vi "Iterate On DB Channels.vi"(8 "error out":errorcluster, 11 "board config handle":u32) -> (0 "error IO":errorcluster, 2 "channels":T1 {"speed" items=["OWL429_HIGH_SPEED_CHANNEL", "OWL429_LOW_SPEED_CHANNEL"]; "Labels"."scheduleBuildUnit" items=["Millisecond", "Microsecond"]}, 3 "board config handle":u32)   [LabVIEW 2016]
uses:
  Controls/AIT_Channel Array.ctl
  Controls/Ballard_Channel.ctl
  Controls/AIT_Label.ctl
  Controls/AIT_Word.ctl
  Controls/ARINCParam.ctl
  Shared/Controls and Global/TransferType.ctl
  Controls/Channel_direction.ctl
  Controls/Channel Speed.ctl
  <userlib>/ARINC-429/Owl429.lvlib
  Ballard Arinc-429 System Explorer.lvlib
  Shared/Ballard Arinc-429 Shared.lvlib
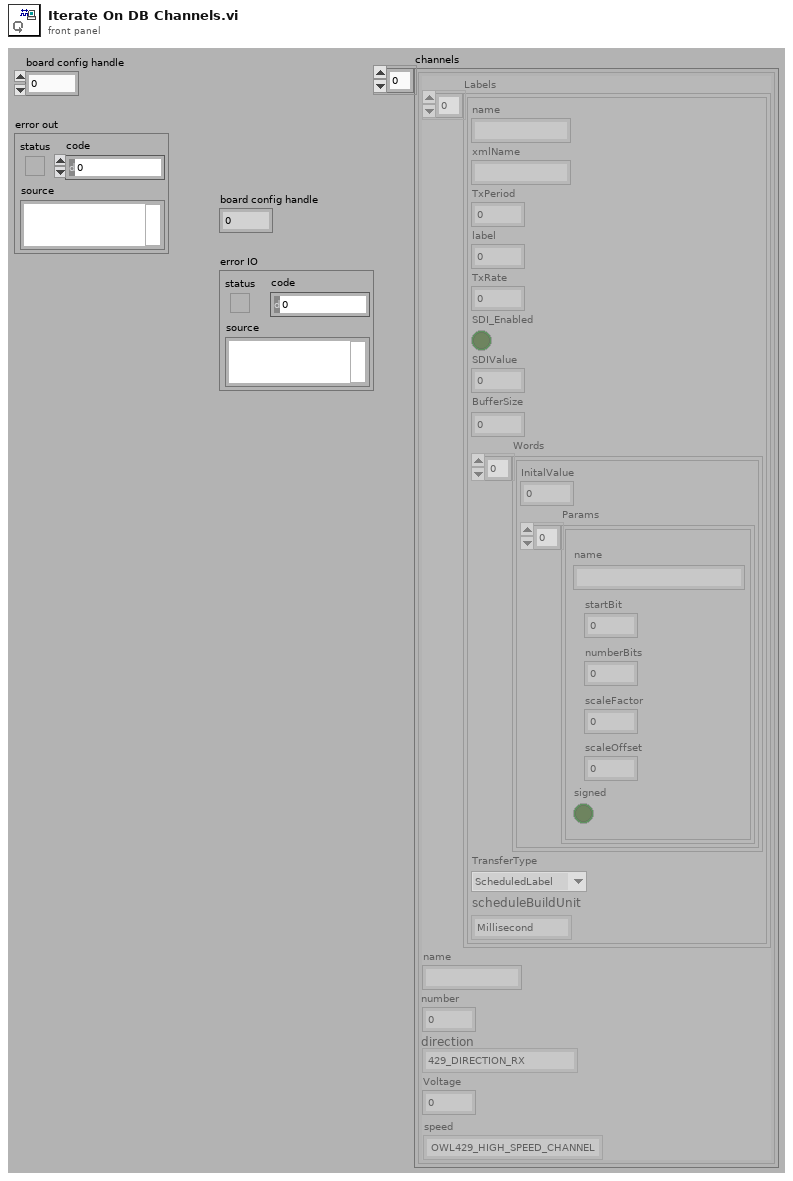
[diagram p1: front panel]
types:
  T1 = typedef "Ballard Arinc-429 System Explorer.lvlib/AIT_Channel Array.ctl" = T2[]
  T2 = typedef "Ballard Arinc-429 System Explorer.lvlib/Ballard_Channel.ctl" = cluster{"Labels":T3[], "name":string, "number":u8, "direction":T7, "Voltage":dbl, "speed":T8}
  T3 = typedef "Ballard Arinc-429 System Explorer.lvlib/AIT_Label.ctl" = cluster{"name":string, "xmlName":string, "TxPeriod":u32, "label":u32, "TxRate":dbl, "SDI_Enabled":bool, "SDIValue":u8, "BufferSize":u32, "Words":T4[], "TransferType":T6, "scheduleBuildUnit":i32}
  T4 = typedef "Ballard Arinc-429 System Explorer.lvlib/AIT_Word.ctl" = cluster{"InitalValue":u32, "Params":T5[]}
  T5 = typedef "Ballard Arinc-429 System Explorer.lvlib/ARINCParam.ctl" = cluster{"name":string, "startBit":i32, "numberBits":i32, "scaleFactor":dbl, "scaleOffset":dbl, "signed":bool}
  T6 = typedef "Ballard Arinc-429 Shared.lvlib/TransferType.ctl" = enum16{"ScheduledLabel", "Acyclic", "Block", "Strobe"}
  T7 = typedef "Channel_direction.ctl" = enum16{"429_DIRECTION_RX", "429_DIRECTION_TX"}
  T8 = typedef "Channel Speed.ctl" = i32
  T9 = enum32{"OWL429_DIRECTION_RX", "OWL429_DIRECTION_TX"}
  T10 = typedef "AIT 429 System Explorer.lvlib/AIT_Channel Array.ctl" = T11[]
  T11 = typedef "AIT 429 System Explorer.lvlib/AIT_Channel.ctl" = cluster{"Labels":T12[], "name":string, "number":u8, "direction":enum16{"OWL429_DIRECTION_RX", "OWL429_DIRECTION_TX"}, "Voltage":dbl, "speed":T16}
  T12 = typedef "AIT 429 System Explorer.lvlib/AIT_Label.ctl" = cluster{"name":string, "xmlName":string, "TxPeriod":u32, "label":u32, "TxRate":dbl, "SDI_Enabled":bool, "SDIValue":u8, "BufferSize":u32, "Words":T13[], "TransferType":T15}
  T13 = typedef "AIT 429 System Explorer.lvlib/AIT_Word.ctl" = cluster{"InitalValue":u32, "Params":T14[]}
  T14 = typedef "AIT 429 System Explorer.lvlib/ARINCParam.ctl" = cluster{"name":string, "startBit":i32, "numberBits":i32, "scaleFactor":dbl, "scaleOffset":dbl, "signed":bool}
  T15 = typedef "ARINC 429 Shared.lvlib/TransferType.ctl" = enum16{"ScheduledLabel", "Acyclic", "Block", "Strobe"}
  T16 = typedef "Owl429.lvlib/Owl429ChannelSpeed.ctl" = enum16{"OWL429_HIGH_SPEED_CHANNEL", "OWL429_LOW_SPEED_CHANNEL"}
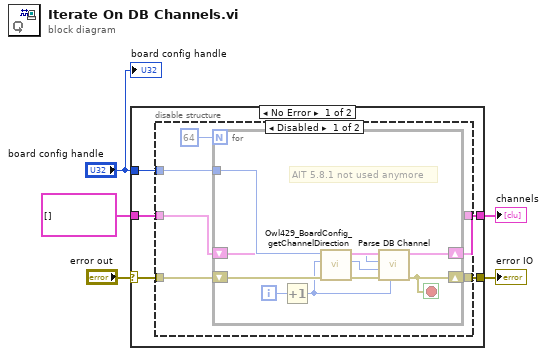
[diagram p0: block diagram]
diagram:
  n1 = case shown="No Error" "error out" {
    selector: "error out" -> [w9 w28]
    tunnel: "board config handle" -> [w6 _]
    tunnel: [w10 w28] -> w2
    tunnel: T1 [] ("channel array") -> [w8 w27]
    tunnel: [w7 w27] -> w5
    frame No Error {
      n2 = disable-structure shown="Disabled" {
        disable-tunnel: [w15 _] -> w10
        disable-tunnel: w9 -> [w14 _]
        disable-tunnel: w8 -> [w13 _]
        disable-tunnel: [w12 _] -> w7
        disable-tunnel: w6 -> [w11 _]
        frame Disabled {
          n3 = for {
            N: 64 -> [_]
            shift-right: [w19] -> w15
            shift-left: w14 -> [w26]
            tunnel: w11 -> [w24]
            shift-right: [w22] -> w12
            shift-left: w13 -> [w23]
            i -> [w25]
            stop <- w19 stop-if-true
            # "AIT 5.8.1 not used anymore"
            n4 = Increment(x=w25) -> (x+1=w21:i32)
            n5 = call <userlib>:"Owl429_BoardConfig_getChannelDirection.vi"("error in (no error)"=w26, "channel number"=w21, "board config handle"=w24) -> ("error out"=w18:errorcluster, "direction"=w20:T9, "board config handle"=w17:u64)  [unwired: 6 in]
            n6 = call "Parse DB Channel.vi"("#"=w21, "error in"=w18, "direction"=w20, "board config handle in"=w17, "Channels"=w23) -> ("error out"=w19:errorcluster, "Channels"=w22:T10)  [unwired: 5 in]
          }
        }
        frame Enabled {
        }
      }
    }
    frame Error {
    }
  }
  "channels" <- w5
  "error IO" <- w2
  "board config handle" <- "board config handle"
